vi "HCC Disable Station Agilent.vi"(8 "Error In":errorcluster, 10 "Raw Input Array":dbl[](array[numeric]), 11 "Disable Channel = True":bool[](array[boolean])) -> (0 "Error Out":errorcluster, 3 "Corrected Array":dbl[](array[numeric]))   [LabVIEW 2016]
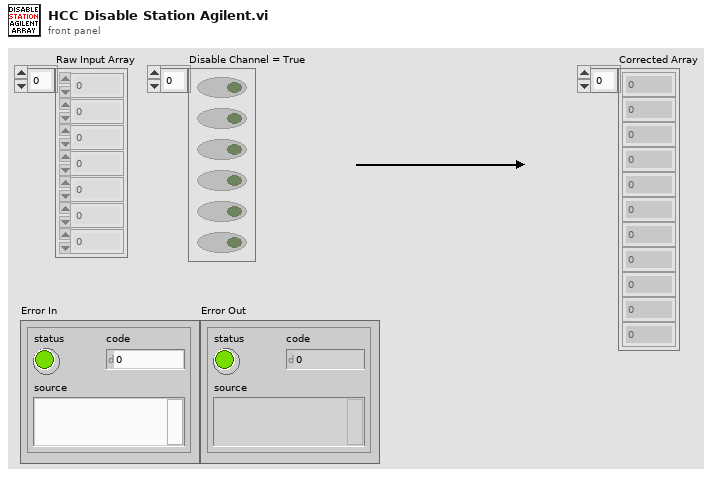
[diagram p1: front panel]
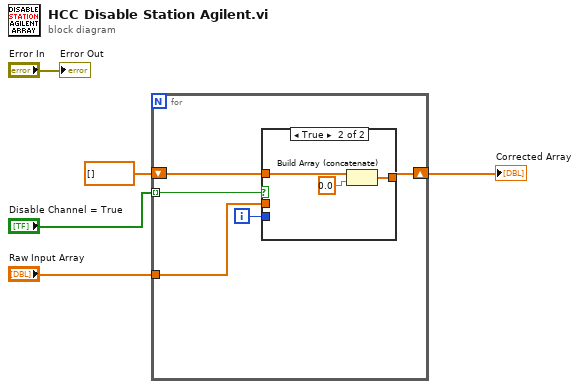
[diagram p0: block diagram]
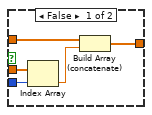
[diagram p2: hidden frame]
diagram:
  n1 = for {
    tunnel: "Disable Channel = True" -> [w10] mode=indexing
    shift-right: [w8] -> w5
    shift-left: dbl[] [] -> [w9]
    tunnel: "Raw Input Array" -> [w7]
    i -> [w6]
    n2 = case shown="True" w10 {
      tunnel: w9 -> [w15 w18]
      tunnel: [w14 w17] -> w8
      tunnel: w6 -> [w11 _]
      tunnel: w7 -> [w12 _]
      frame False {
        n3 = Index Array(array=w12, index=w11) -> (element=w13:dbl)
        n4 = Build Array (concatenate)(w15, w13) -> (w14:dbl[])
      }
      frame True {
        n5 = Build Array (concatenate)(w18, 0.0) -> (w17:dbl[])
      }
    }
  }
  "Corrected Array" <- w5
  "Error Out" <- "Error In"
